vi "Color to ColorBox.vi"(8 "error in (no error)":errorcluster caption="错误输入（无错误）", 11 "Color":refnum<k24>) -> (0 "error out":errorcluster caption="错误输出", 3 "ColorBox":u32(colorbox))   [LabVIEW 2012, in "Color.lvclass"]
uses:
  Color.lvclass
  System.Drawing
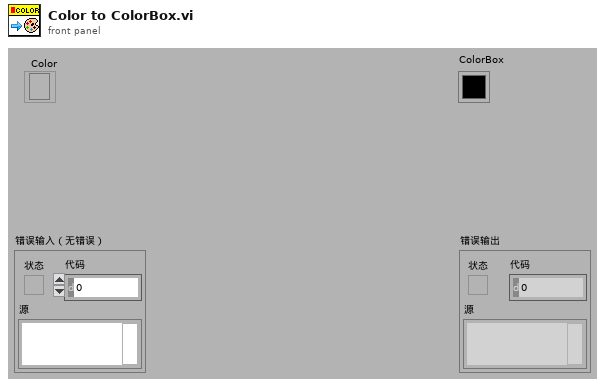
[diagram p1: front panel]
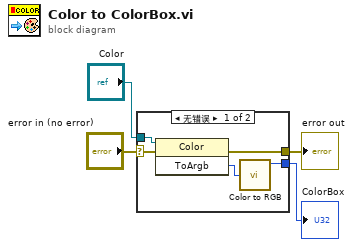
[diagram p0: block diagram]
diagram:
  n1 = case shown="无错误" "error in (no error)" {
    selector: "error in (no error)" -> [w9 w10]
    tunnel: [w8 w10] -> w3
    tunnel: [w7 _] -> w2
    tunnel: "Color" -> [w5 _]
    frame No Error {
      n2 = invoke class="Color" method="ToArgb"(reference=w5, error in=w9) -> (error out=w8:errorcluster, "ToArgb"=w6:i32)  [unwired: 1 in, 1 out]
      n3 = call <vilib>:"Color to RGB.vi"("Color"=w6) -> ("Resolved Color"=w7:u32)  [unwired: 3 out]
    }
    frame Error {
    }
  }
  "error out" <- w3
  "ColorBox" <- w2
